vi "Connect TCP.vi"(6 "timeout (100ms)":i32=100, 8 "error in (no error)":errorcluster, 10 "remote port (80)":u16=80, 11 "address (localhost)":string="localhost") -> (0 "error out":errorcluster, 3 "TCPConnection out":refnum<class "TCPConnection.lvclass">)   [LabVIEW 2013, in "MQTT Server.lvlib" / "TCPConnection.lvclass"]
uses:
  TCPConnection.lvclass
  connection notifier.ctl
  TCPConnection.lvclass/TCPConnection.ctl
  connection_process.vi
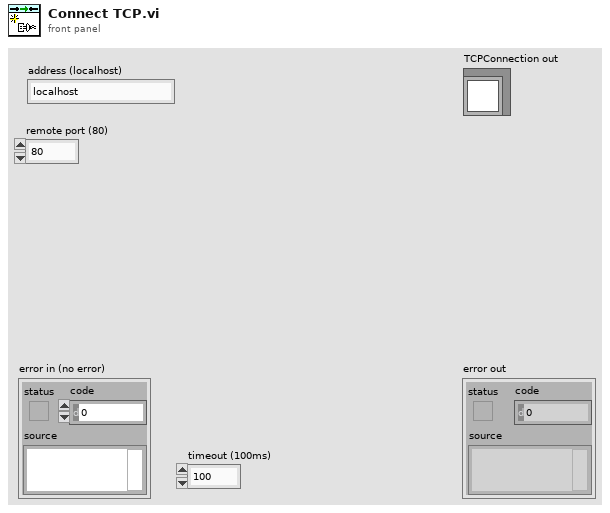
[diagram p1: front panel]
types:
  T1 = typedef "MQTT Server.lvlib/TCPConnection.lvclass/connection notifier.ctl" = cluster{"connection ID":refnum<k5>, "error IO":errorcluster}
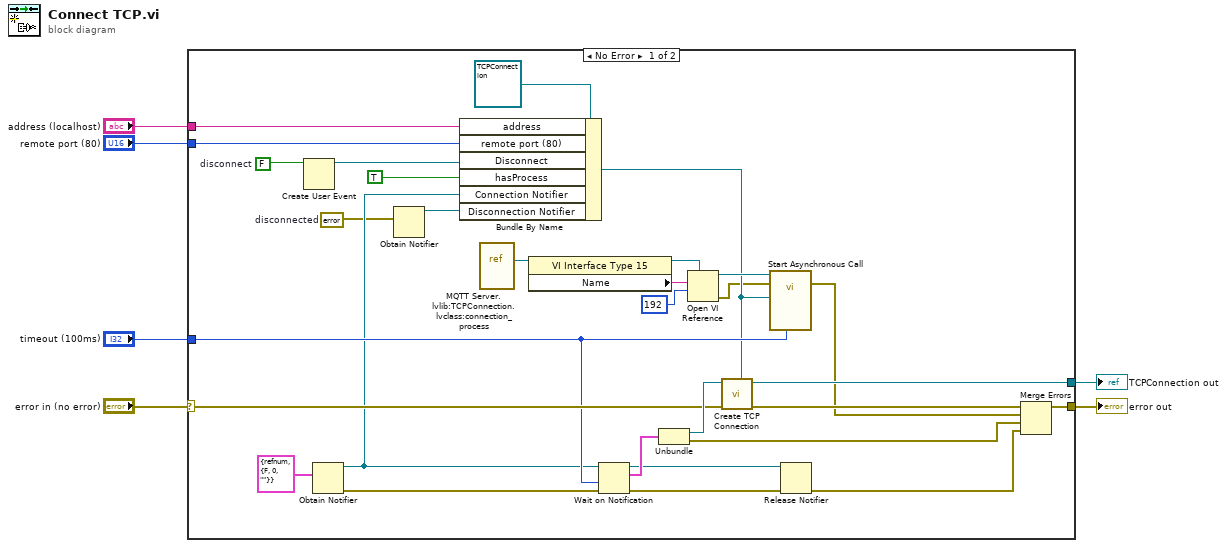
[diagram p0: block diagram]
diagram:
  n1 = case shown="No Error" "error in (no error)" {
    selector: "error in (no error)" -> [w30 w37]
    tunnel: [w31 w37] -> w5
    tunnel: [w18 _] -> w4
    tunnel: "address (localhost)" -> [w20 _]
    tunnel: "remote port (80)" -> [w19 _]
    tunnel: "timeout (100ms)" -> [w25 _]
    frame No Error {
      w7 = errorcluster {"status"=FALSE, "code"=0, "source"=""}  # disconnected
      w23 = FALSE  # disconnect
      n2 = Create User Event(user event datatype=w23) -> (user event=w22:refnum<user-event>)  [unwired: 1 in, 1 out]
      n3 = Obtain Notifier(notification data type=T1 {"connection ID"=refnum, "error IO"={"status"=FALSE, "code"=0, "source"=""}} ("MQTT Server.lvlib:TCPConnection.lvclass:connection notifier")) -> (notifier out=w16:refnum<notifier>, error out=w36:errorcluster)  [unwired: 3 in, 1 out]
      n4 = Obtain Notifier(notification data type=w7) -> (notifier out=w14:refnum<notifier>)  [unwired: 3 in, 2 out]
      n5 = Bundle By Name(cluster=refnum<class "TCPConnection.lvclass"> refnum ("TCPConnection in"), "address"=w20, "remote port (80)"=w19, "Disconnect"=w22, "hasProcess"=TRUE, "Connection Notifier"=w16, "Disconnection Notifier"=w14) -> (w10:refnum<class "TCPConnection.lvclass">)
      n6 = vi-ref "MQTT Server.lvlib:TCPConnection.lvclass:connection_process.vi"() -> (w29:refnum<vi>)
      n7 = property class="VI Interface Type 15"(reference=w29) -> (reference out=w27:refnum<vi>, "Name"=w28:string)  [unwired: 1 in, 1 out]
      n8 = Wait on Notification(notifier=w16, timeout in ms (-1)=w25, error in (no error)=w36) -> (notifier out=w11:refnum<notifier>, notification=w35:T1, error out=w13:errorcluster)  [unwired: 1 in, 1 out]
      n9 = Unbundle(w35) -> ("connection ID"=w34:refnum<k5>, "error IO"=w33:errorcluster)
      n10 = Open VI Reference(type specifier VI Refnum (for type only)=w27, vi path=w28, options=192) -> (vi reference=w26:refnum<vi>, error out=w8:errorcluster)  [unwired: 3 in]
      n11 = call "Create TCP Connection.vi"("TCPConnection in"=w10, "error in (no error)"=w30, "connection ID"=w34) -> ("error out"=w32:errorcluster, "TCPConnection out"=w18:refnum<class "TCPConnection.lvclass">)  [unwired: 7 in]
      n12 = call-by-ref "Start Asynchronous Call"(reference=w26, error in=w8, "timeout (ms)"=w25, "TCPConnection"=w10) -> (error out=w9:errorcluster)  [unwired: 10 in, 1 out]
      n13 = Release Notifier(notifier=w11, error in (no error)=w13) -> (error out=w12:errorcluster)  [unwired: 1 in, 2 out]
      n14 = Merge Errors(w32, w9, w33, w12) -> (w31:errorcluster)
    }
    frame Error {
    }
  }
  "error out" <- w5
  "TCPConnection out" <- w4
